vi "Obis Test Panel.vi"() -> ()   [LabVIEW 2020]
uses:
  <vilib>/Instr/_visa.llb/VISA Configure Serial Port (Instr).vi
panel:
  out "Response":string
  in  "Quit":bool
  in  "Send Command":bool
  in  "Command":string
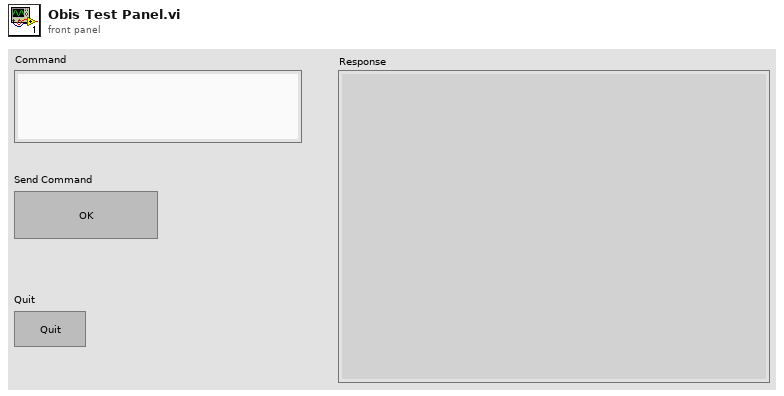
[diagram p1: front panel]
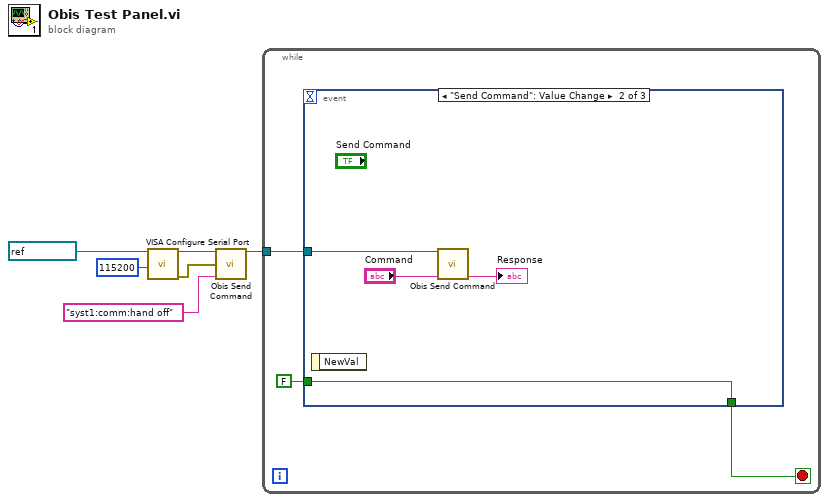
[diagram p0: block diagram]
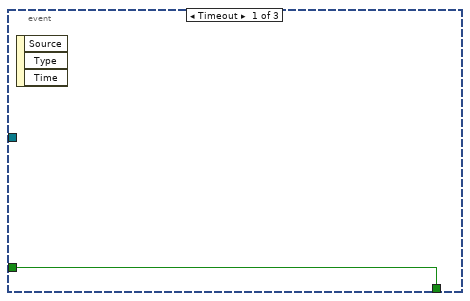
[diagram p2: hidden frame]
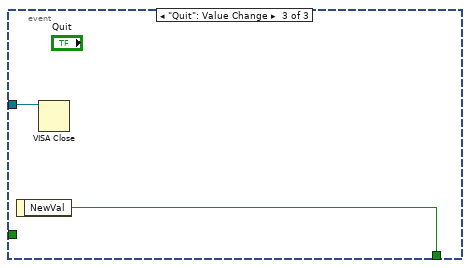
[diagram p3: hidden frame]
diagram:
  n1 = call-poly "VISA Configure Serial Port"("VISA resource name"=refnum<visa-resource-name> "COM11" ("reference"), "baud rate (9600)"=u32 115200) -> ("VISA resource name out"=w4:refnum<visa-resource-name>, "error out"=w1:errorcluster)  [unwired: 12 in]
  n2 = call "Obis Send Command.vi"("VISA Ref"=w4, "Error In"=w1, "Command"="syst1:comm:hand off" ("write to laser")) -> ("VISA Ref Out"=w3:refnum<visa-resource-name>)  [unwired: 10 in, 2 out]
  n3 = while {
    tunnel: w3 -> [w7]
    stop <- w9 stop-if-true
    n4 = event shown="[1] \"Send Command\": Value Change" {
      selector: _ -> [_ _ _]
      dyn-events: _ -> [_ _ _]
      timeout: _ -> [_ _ _]
      tunnel: [w10 w14 w16] -> w9
      tunnel: FALSE -> [w10 w14 _]
      tunnel: w7 -> [_ w13 w15]
      event Timeout {
        n5 = event-data() -> ()  [unwired: 1 in, 3 out]
      }
      event "Send Command": Value Change {
        n6 = event-data() -> ()  [unwired: 1 in, 1 out]
        n7 = call "Obis Send Command.vi"("VISA Ref"=w13, "Command"="Command") -> ("Response"=→"Response":string)  [unwired: 11 in, 2 out]
      }
      event "Quit": Value Change {
        n8 = event-data() -> ("NewVal"=w16:bool)  [unwired: 1 in]
        n9 = VISA Close(VISA resource name=w15) -> ()  [unwired: 1 in, 1 out]
      }
    }
  }
